vi "modbusw.vi"(0 "TCP master instance":refnum<class "Modbus Master.lvclass">, 1 "D0":bool, 2 "D1":bool, 3 "D2":bool, 7 "starting addres":u16 step=5, 11 "Error In":errorcluster, 12 "D3":bool, 13 "D4":bool) -> (4 "Modbus master out":refnum<class "Modbus Master.lvclass">, 15 "error out":errorcluster)   [LabVIEW 2019]
uses:
  <vilib>/NI/Modbus Library/API/Master/Modbus Master.lvclass
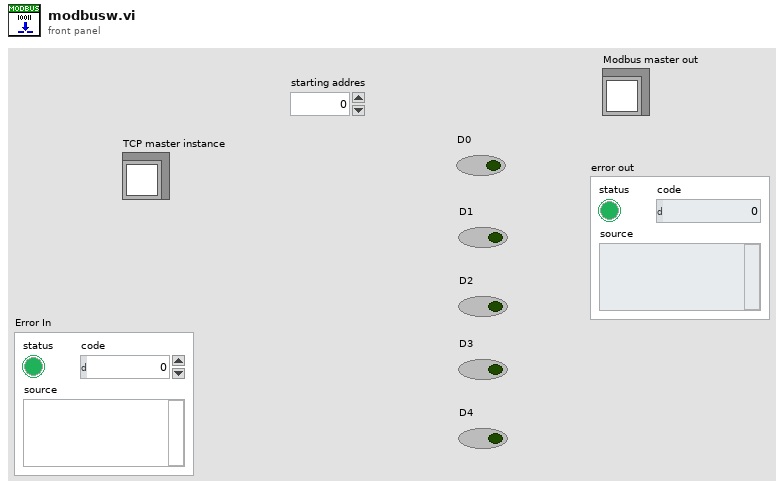
[diagram p1: front panel]
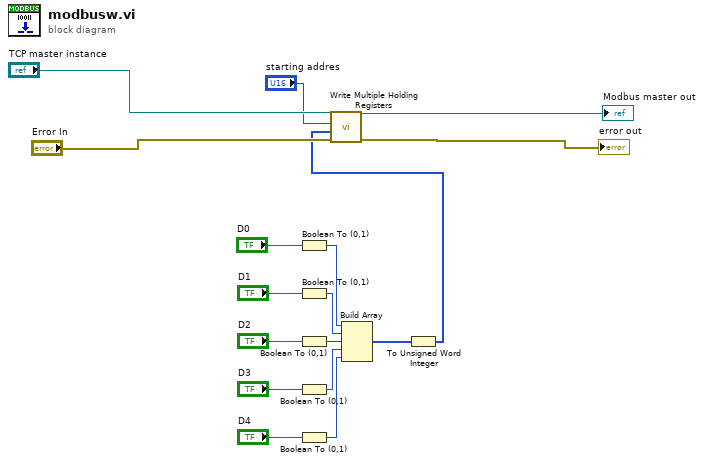
[diagram p0: block diagram]
diagram:
  n1 = Boolean To (0,1)(Boolean="D0") -> (0, 1=w8:i16)
  n2 = Boolean To (0,1)(Boolean="D1") -> (0, 1=w9:i16)
  n3 = Boolean To (0,1)(Boolean="D2") -> (0, 1=w10:i16)
  n4 = Boolean To (0,1)(Boolean="D3") -> (0, 1=w11:i16)
  n5 = Boolean To (0,1)(Boolean="D4") -> (0, 1=w12:i16)
  n6 = Build Array(w8, w9, w10, w11, w12) -> (w13:i16[])
  n7 = To Unsigned Word Integer(number=w13) -> (unsigned 16bit integer=w2:u16[])
  n8 = call-dynamic "Write Multiple Holding Registers.vi"("error in"="Error In", "registers to write"=w2, "starting address"="starting addres", "Modbus master in"="TCP master instance") -> ("error out"=→"error out":errorcluster, "Modbus master out"=→"Modbus master out":refnum<class "Modbus Master.lvclass">)  [unwired: 6 in]
